vi "Create Real Matrix From Eigenvalues.vi"(3 "Eigenvalues":cdb[](array[numeric]) format="%.2f") -> (0 "error":i32, 1 "Matrix":T1)   [LabVIEW 2017, in "NI_AALPro.lvlib"]
doc: "Generates a real matrix from <B>Eigenvalues</B>."
uses:
  NI_AALPro.lvlib
  RealMatrix.ctl
  <resource>/lvanlys.dll
  NI_Matrix.lvlib
panel:
  # "Create Real Matrix From Eigenvalues"
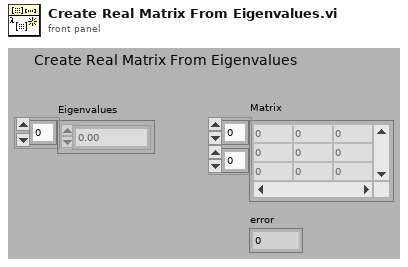
[diagram p1: front panel]
types:
  T1 = typedef "NI_Matrix.lvlib/RealMatrix.ctl" = dbl[][]
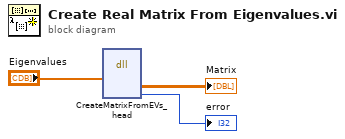
[diagram p0: block diagram]
diagram:
  n1 = dll-call lib="C:/Program Files (x86)/National Instruments/LabVIEW 2017/resource/lvanlys.*" fn="CreateMatrixFromEVs_head"("Eigenvalues"="Eigenvalues") -> ("Matrix"=→"Matrix":T1, "error"=→"error":i32)  [unwired: 7 in, 2 out]
